vi "Write Data.vi"(8 "error in (no error)":errorcluster, 9 "Publication Time":timestamp, 10 "Value":variant, 11 "TerminalVisibilityBinding In":refnum<class "TerminalVisibilityBinding.lvclass">) -> (0 "error out":errorcluster, 3 "TerminalVisibilityBinding Out":refnum<class "TerminalVisibilityBinding.lvclass">)   [LabVIEW 2015, in "Transport.lvlib" / "TerminalVisibilityBinding.lvclass"]
doc: "<License>\nCopyright © 2017 Composed Systems, LLC | All rights reserved\nwww.composed.io\n\nAuthor: Ethan Stern <ethan.stern@composed.io>\n\nThis software is provided \"AS IS\" WITHOUT WARRANTIES, either express or implied, AND IS FOR EDUCATIONAL PURPOSES ONLY.\n</License>"
uses:
  TerminalVisibilityBinding.lvclass
  TerminalVisibilityBinding.lvclass/TerminalVisibilityBinding.ctl
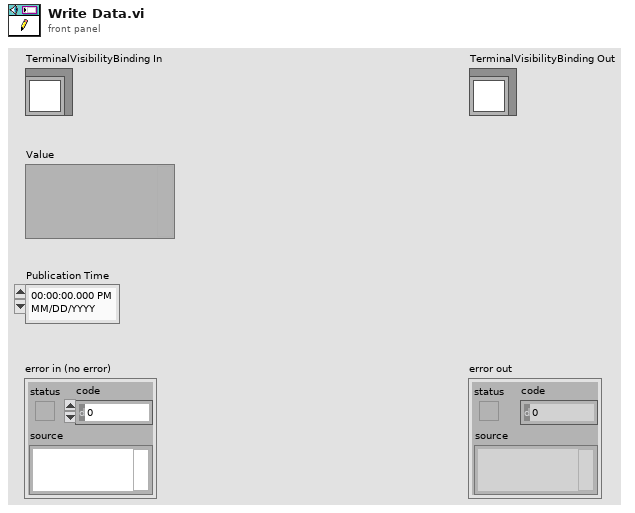
[diagram p1: front panel]
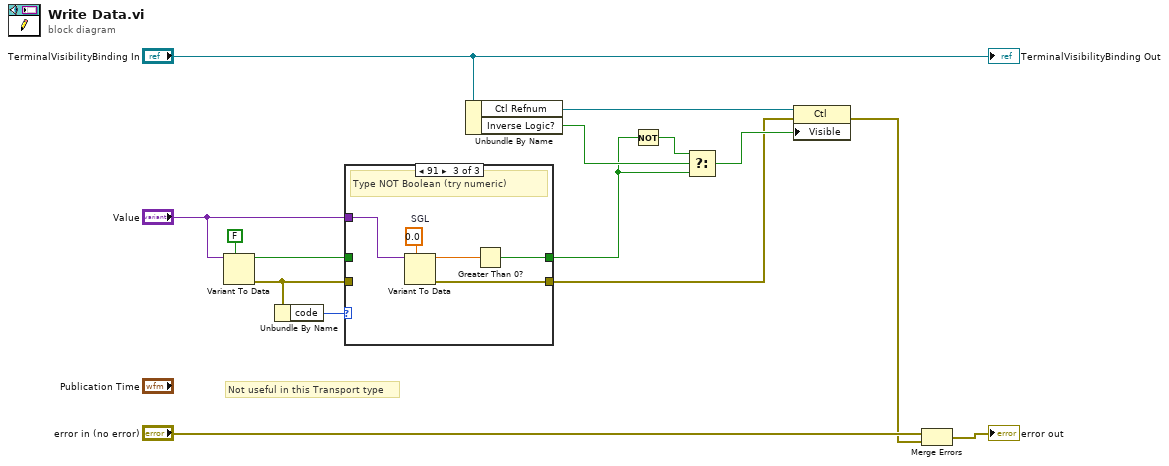
[diagram p0: block diagram]
diagram:
  # "Not useful in this Transport type"
  n1 = Variant To Data(type=FALSE, Variant="Value") -> (data=w5:bool, error out=w3:errorcluster)  [unwired: 1 in]
  n2 = Unbundle By Name(w3) -> ("code"=w6:i32)
  n3 = case shown="91" w6 {
    tunnel: w5 -> [w17 w19 _]
    tunnel: [w17 w19 w22] -> w4
    tunnel: "Value" -> [_ _ w21]
    tunnel: [w16 w18 w20] -> w2
    tunnel: w3 -> [w16 w18 _]
    frame Default {
      # "A more serious (unexpected) error"
    }
    frame 0 {
      # "Type = Boolean (OK)"
    }
    frame 91 {
      w24 = sgl 0.0  # SGL
      # "Type NOT Boolean (try numeric)"
      n4 = Variant To Data(type=w24, Variant=w21) -> (data=w23:sgl, error out=w20:errorcluster)  [unwired: 1 in]
      n5 = Greater Than 0?(x=w23) -> (x > 0?=w22:bool)
    }
  }
  n6 = Unbundle By Name("TerminalVisibilityBinding In") -> ("Ctl Refnum"=w13:refnum<vi>, "Inverse Logic?"=w9:bool)
  n7 = Not(x=w4) -> (.not. x?=w7:bool)
  n8 = Select(t=w7, s=w9, f=w4) -> (s? t:f=w8:bool)
  n9 = property class="Ctl"(reference=w13, error in=w2, "Visible"=w8) -> (error out=w11:errorcluster)  [unwired: 1 out]
  n10 = Merge Errors("error in (no error)", w11) -> (→"error out":errorcluster)
  "TerminalVisibilityBinding Out" <- "TerminalVisibilityBinding In"
